vi "Test Base Persist Arguments from Init.vi"(8 "error in (no error)":errorcluster, 11 "Base Class Test In":refnum<class "Base Test.lvclass">) -> (0 "error out":errorcluster, 3 "Base Class Test Out":refnum<class "Base Test.lvclass">)   [LabVIEW 2020, in "Base Test.lvclass"]
uses:
  Base Test.lvclass
  C:/Program Files (x86)/National Instruments/LabVIEW 2020/vi.lib/Asteme/LUnit/Test Case.lvclass
  Base Test.lvclass/Base Test.ctl
  Framework/Base/Base.lvclass/Base.ctl
  <vilib>/Asteme/LUnit/Test Case.lvclass/Test Case.ctl
  <vilib>/Asteme/LUnit/LUnit Assertion Result.lvclass/LUnit Assertion Result.ctl
  <vilib>/Asteme/LUnit/Palette/Pass.vi
  <vilib>/Asteme/LUnit/Palette/Fail.vi
  <vilib>/Asteme/LUnit/Variant to string.vi
  <vilib>/Asteme/LUnit/Set Assertion Type.vi
  <vilib>/Asteme/LUnit/Add test result.vi
  <vilib>/Asteme/LUnit/LUnit Write Passed.vi
  <vilib>/Asteme/LUnit/LUnit Get Test Case.vi
  <vilib>/Asteme/LUnit/Assertion Result/LUnit Get Test Name.vi
  <vilib>/Asteme/LUnit/LUnit Write Message.vi
  <vilib>/Asteme/LUnit/LUnit Write Description.vi
  <vilib>/Asteme/LUnit/LUnit Write Assertion Type.vi
  <vilib>/Asteme/LUnit/Read Test Case Name.vi
  <vilib>/Utility/Data Type/Get Type Information.vi
  <vilib>/Utility/LVClass/Get LV Class Name.vi
  Framework/Base/Base.lvclass
  <vilib>/Asteme/LUnit/LUnit Assertion Result.lvclass
  <vilib>/Asteme/LUnit/Test Case.lvclass
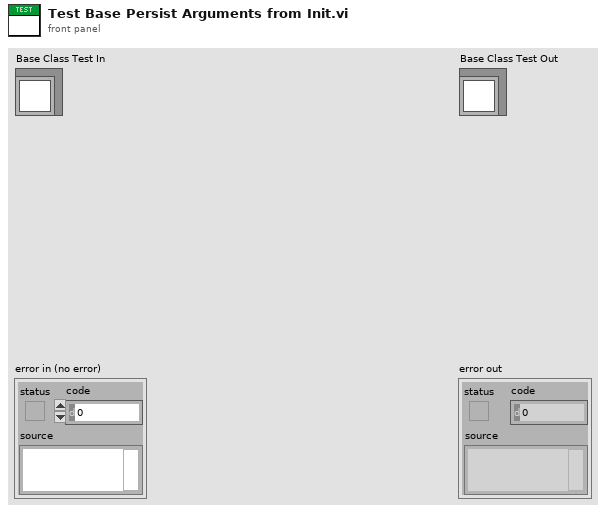
[diagram p1: front panel]
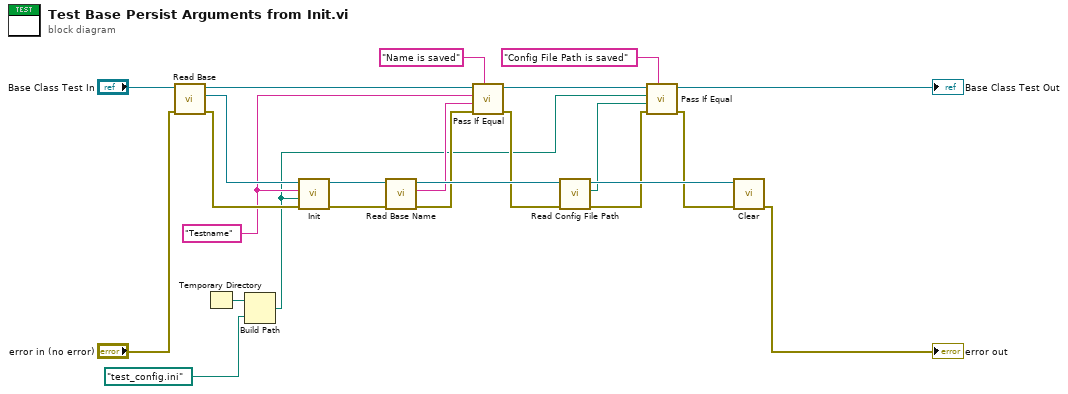
[diagram p0: block diagram]
diagram:
  w14 = "Testname" ("Name")
  n1 = call "Read Base.vi"("error in (no error)"="error in (no error)", "Base Class Test In"="Base Class Test In") -> ("error out"=w16:errorcluster, "Base.lvclass"=w18:refnum<class "Base.lvclass">, "Base Class Test Out"=w19:refnum<class "Base Test.lvclass">)  [unwired: 7 in]
  n2 = Temporary Directory() -> (w3:path)
  n3 = Build Path(base path=w3, name or relative path=path "test_config.ini" ("Config File Path")) -> (appended path=w2:path)
  n4 = call-dynamic "Init.vi"("error in (no error)"=w16, "Config File Path"=w2, "Name"=w14, "Base In"=w18) -> ("error out"=w22:errorcluster, "Base Out"=w23:refnum<class "Base.lvclass">)  [unwired: 6 in]
  n5 = call-dynamic "Read Base Name.vi"("error in (no error)"=w22, "Base In"=w23) -> ("error out"=w12:errorcluster, "Name"=w13:string, "Base Out"=w21:refnum<class "Base.lvclass">)  [unwired: 7 in]
  n6 = call <vilib>:"Pass If Equal.vi"("Description"="Name is saved", "error in (no error)"=w12, "Actual"=w13, "Expected"=w14, "Test Case In"=w19) -> ("error out"=w11:errorcluster, "Test Case Out"=w15:refnum<class "Base Test.lvclass">)  [unwired: 5 in]
  n7 = call "Read Config File Path.vi"("error in (no error)"=w11, "Process In"=w21) -> ("error out"=w9:errorcluster, "Config File Path"=w10:path, "Process Out"=w20:refnum<class "Base.lvclass">)  [unwired: 7 in]
  n8 = call <vilib>:"Pass If Equal.vi"("Description"="Config File Path is saved", "error in (no error)"=w9, "Actual"=w10, "Expected"=w2, "Test Case In"=w15) -> ("error out"=w8:errorcluster, "Test Case Out"=→"Base Class Test Out":refnum<class "Base Test.lvclass">)  [unwired: 5 in]
  n9 = call-dynamic "Clear.vi"("error in (no error)"=w8, "Base In"=w20) -> ("error out"=→"error out":errorcluster)  [unwired: 9 in]
